vi "Elevator Manual Control 2.0.vi"(9 "Down":bool, 10 "Up":bool, 11 "Enabled":bool) -> ()   [LabVIEW 2014]
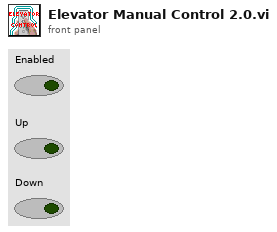
[diagram p1: front panel]
types:
  T1 = typedef "WPI_PotentiometerDevRef.ctl" = cluster{"DevStatus":errorcluster, "Controller":T2, "Analog Channel":T3, "Invert Output":bool}
  T2 = typedef "FPGA_TypedefAnalogModule.ctl" = enum16{"Controller 1"}
  T3 = typedef "FPGA_AIChannel.ctl" = enum8{"AI 0", "AI 1", "AI 2", "AI 3", "AI MXP 0", "AI MXP 1", "AI MXP 2", "AI MXP 3", "Invalid"}
  T4 = typedef "WPI_MotorControlDeviceRef.ctl" = cluster{"DeviceStatus":errorcluster, "Type":T5, "PWM":cluster{"Controller":T6, "PWM Channel":T7, "DeadBand":T8}, "CAN":cluster{"Device Number":u8, "Control Mode":T9, "Semaphore":T10, "Max Vout":dbl, "TalonSRX Control Mode":T11}, "Invert":bool, "TransformRef":T12, "InvTransformRef":T12}
  T5 = typedef "WPI_MotorControlType.ctl" = enum16{"PWM", "CAN", "CANTalonSRX"}
  T6 = typedef "FPGA_TypedefDigitalModule.ctl" = enum16{"Controller 1"}
  T7 = typedef "FPGA_DIOPWMChannel.ctl" = enum8{"PWM 0", "PWM 1", "PWM 2", "PWM 3", "PWM 4", "PWM 5", "PWM 6", "PWM 7", "PWM 8", "PWM 9", "PWM MXP 0", "PWM MXP 1", "PWM MXP 2", "PWM MXP 3", "PWM MXP 4", "PWM MXP 5", "PWM MXP 6", "PWM MXP 7", "PWM MXP 8", "PWM MXP 9", "Invalid"}
  T8 = typedef "WPI_PWMDeadband.ctl" = cluster{"Name":string, "maxPositivePwm":i32, "minPositivePwm":i32, "centerPwm":i32, "maxNegativePwm":i32, "minNegativePwm":i32, "angularRange":u16}
  T9 = typedef "WPI_CANJaguar_ControlMode.ctl" = enum8{"Percent VBus", "Current", "Speed", "Position", "Voltage"}
  T10 = typedef "Semaphore RefNum" = refnum<k1>
  T11 = typedef "WPI_CANTalonSRX_APIControlMode.ctl" = enum8{"Percent VBus", "Speed", "Position", "Slave", "Unchanged / Invalid"}
  T12 = typedef "WPI_PWMTransform_ConPane.ctl" = refnum<vi>
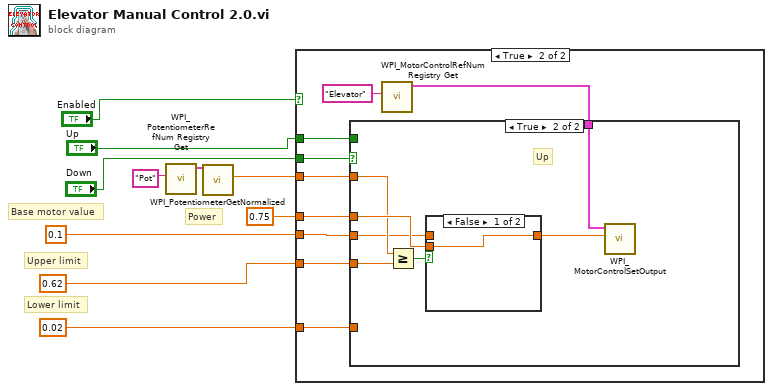
[diagram p0: block diagram]
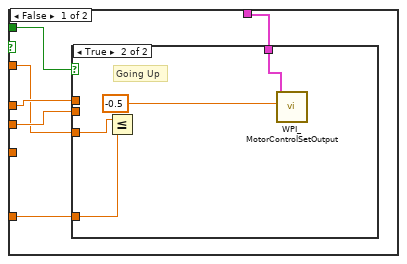
[diagram p3: hidden frame]
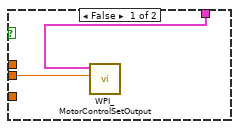
[diagram p4: hidden frame]
diagram:
  # "Power"
  # "Lower limit"
  # "Upper limit"
  # "Base motor value"
  n1 = call <vilib>:"WPI_PotentiometerRefNum Registry Get.vi"("refnum name"="Pot") -> ("PotDevRef"=w1:T1)  [unwired: 9 in, 1 out]
  n2 = call <vilib>:"WPI_PotentiometerGetNormalized.vi"("PotDevRef"=w1) -> ("Normalized Value"=w4:dbl)  [unwired: 8 in, 2 out]
  n3 = case shown="True" "Enabled" {
    tunnel: "Down" -> [_ w17]
    tunnel: "Up" -> [_ w16]
    tunnel: 0.1 ("Output") -> [_ w15]
    tunnel: 0.75 ("Output") -> [_ w14]
    tunnel: w4 -> [_ w13]
    tunnel: 0.62 ("Output") -> [_ w12]
    tunnel: 0.02 ("Output") -> [_ w11]
    frame False {
    }
    frame True {
      n4 = call <vilib>:"WPI_MotorControlRefNum Registry Get.vi"("refnum name"="Elevator") -> ("MotorControlDevRef"=w19:T4)  [unwired: 9 in, 1 out]
      n5 = case shown="True" w17 {
        tunnel: w19 -> [w25 w38]
        tunnel: w16 -> [w24 _]
        tunnel: w15 -> [w23 w32]
        tunnel: w14 -> [w22 w36]
        tunnel: w13 -> [w21 w34]
        tunnel: w12 -> [_ w33]
        tunnel: w11 -> [w20 _]
        frame False {
          n6 = case shown="True" w24 {
            tunnel: w25 -> [w27 w31]
            tunnel: w23 -> [w26 _]
            tunnel: w22 -> [_ _]
            tunnel: w21 -> [_ w30]
            tunnel: w20 -> [_ w29]
            frame False {
              n7 = call <vilib>:"WPI_MotorControlSetOutput.vi"("Output"=w26, "MotorControlDevRef"=w27) -> ()  [unwired: 7 in, 3 out]
            }
            frame True {
              # "Going Up"
              n8 = Less Or Equal?(x=w30, y=w29) -> ()  [unwired: 1 out]
              n9 = call <vilib>:"WPI_MotorControlSetOutput.vi"("Output"=-0.5, "MotorControlDevRef"=w31) -> ()  [unwired: 7 in, 3 out]
            }
          }
        }
        frame True {
          # "Up"
          n10 = Greater Or Equal?(x=w34, y=w33) -> (x >= y?=w35:bool)
          n11 = case shown="False" w35 {
            tunnel: [w39 w40] -> w37
            tunnel: w36 -> [w39 _]
            tunnel: w32 -> [_ w40]
            frame False {
            }
            frame True {
            }
          }
          n12 = call <vilib>:"WPI_MotorControlSetOutput.vi"("Output"=w37, "MotorControlDevRef"=w38) -> ()  [unwired: 7 in, 3 out]
        }
      }
    }
  }
